vi "Update Refs.vi"(8 "error in (no error)":errorcluster, 10 "SequencerInfo":refnum<class "SequencerInfo.lvclass">, 11 "UI in":refnum<class "UI.lvclass">) -> (0 "error out":errorcluster, 3 "UI out":refnum<class "UI.lvclass">)   [LabVIEW 2015, in "UI.lvlib" / "UI.lvclass"]
uses:
  UI.lvclass
  Sequencer/SequencerInfo.lvclass
  Sequencer/SequencerConfig.lvclass
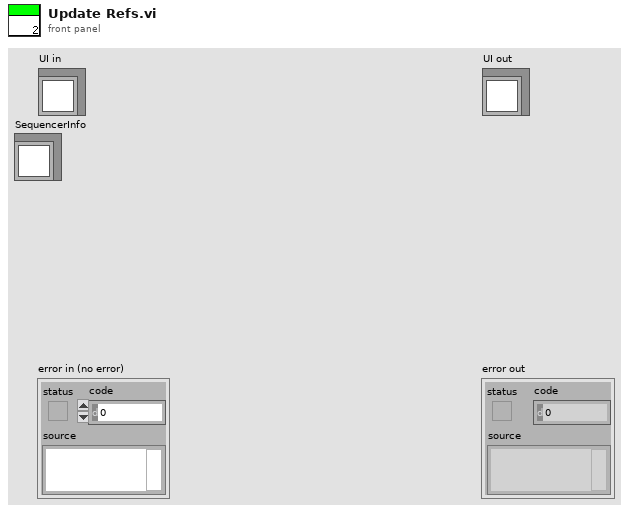
[diagram p1: front panel]
types:
  T1 = typedef "Sequencer.lvlib/Sequencer.lvclass/Daq Channel Info.ctl" = cluster{"DevNames":tag[], "AO.PhysicalChans":tag[][], "DO.Lines":tag[][], "AI.PhysicalChans":tag[][]}
  T2 = cluster{"Accessors:Sample Rate":dbl, "Accessors:Buffer Size":dbl}
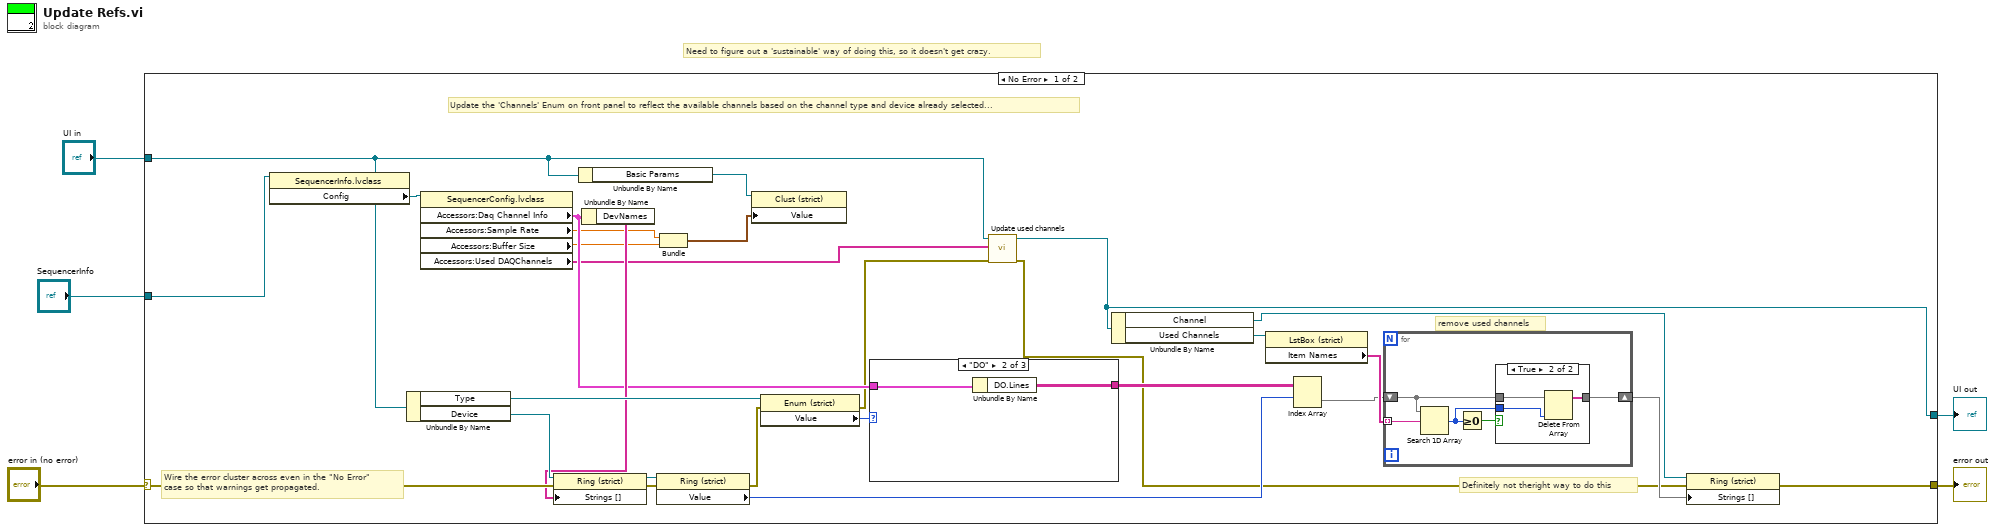
[diagram p0: block diagram]
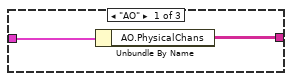
[diagram p3: hidden frame]
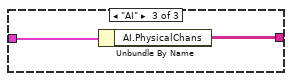
[diagram p4: hidden frame]
diagram:
  # "Need to figure out a 'sustainable' way of doing this, so it doesn't get crazy."
  n1 = case shown="No Error" "error in (no error)" {
    selector: "error in (no error)" -> [w25 w50]
    tunnel: [w14 w50] -> w4
    tunnel: [w8 w49] -> w2
    tunnel: "UI in" -> [w9 w49]
    tunnel: "SequencerInfo" -> [w11 _]
    frame No Error {
      # "Update the 'Channels' Enum on front panel to reflect the available channels based on the channel type and device already selected..."
      # "remove used channels"
      # "Definitely not theright way to do this"
      # "Wire the error cluster across even in the \"No Error\"\ncase so that warnings get propagated."
      n2 = property class="SequencerInfo.lvclass"(reference=w11) -> ("Config"=w19:refnum<class "SequencerConfig.lvclass">)  [unwired: 1 in, 2 out]
      n3 = Unbundle By Name(w9) -> ("Type"=w30:refnum<vi>, "Device"=w33:refnum<vi>)
      n4 = property class="SequencerConfig.lvclass"(reference=w19) -> ("Accessors:Daq Channel Info"=w17:T1, "Accessors:Sample Rate"=w16:dbl, "Accessors:Buffer Size"=w15:dbl, "Accessors:Used DAQChannels"=w10:tag[])  [unwired: 1 in, 2 out]
      n5 = Unbundle By Name(w9) -> ("Basic Params"=w13:refnum<vi>)
      n6 = Unbundle By Name(w17) -> ("DevNames"=w18:tag[])
      n7 = property class="Ring (strict)"(reference=w33, error in=w25, "Strings []"=w18) -> (reference out=w32:refnum<vi>, error out=w31:errorcluster)
      n8 = property class="Ring (strict)"(reference=w32, error in=w31) -> (error out=w26:errorcluster, "Value"=w24:u16)  [unwired: 1 out]
      n9 = Bundle("Accessors:Sample Rate"=w16, "Accessors:Buffer Size"=w15) -> (w12:T2)  [unwired: 1 in]
      n10 = property class="Clust (strict)"(reference=w13, "Value"=w12) -> ()  [unwired: 1 in, 2 out]
      n11 = property class="Enum (strict)"(reference=w30, error in=w26) -> (error out=w7:errorcluster, "Value"=w29:enum16{"AO", "DO", "AI"})  [unwired: 1 out]
      n12 = case shown="\"DO\"" w29 {
        tunnel: [w44 w46 w48] -> w27
        tunnel: w17 -> [w43 w45 w47]
        frame "AO" {
          n13 = Unbundle By Name(w43) -> ("AO.PhysicalChans"=w44:tag[][])
        }
        frame "DO" {
          n14 = Unbundle By Name(w45) -> ("DO.Lines"=w46:tag[][])
        }
        frame "AI" {
          n15 = Unbundle By Name(w47) -> ("AI.PhysicalChans"=w48:tag[][])
        }
      }
      n16 = call "Update used channels.vi"("error in (no error)"=w7, "Used DAQ Channels in"=w10, "UI in"=w9) -> ("error out"=w6:errorcluster, "UI out"=w8:refnum<class "UI.lvclass">)  [unwired: 7 in]
      n17 = Unbundle By Name(w8) -> ("Channel"=w28:refnum<vi>, "Used Channels"=w23:refnum<vi>)
      n18 = property class="LstBox (strict)"(reference=w23) -> ("Item Names"=w22:string[])  [unwired: 1 in, 2 out]
      n19 = Index Array(array=w27, index (row)=w24) -> (element=w21:tag[])  [unwired: 1 in]
      n20 = for {
        tunnel: w22 -> [w38] mode=indexing
        shift-right: [w36] -> w20
        shift-left: w21 -> [w37]
        n21 = Search 1D Array(1D array=w37, element=w38) -> (index of element=w35:i32)  [unwired: 1 in]
        n22 = Greater Or Equal To 0?(x=w35) -> (x >= 0?=w34:bool)
        n23 = case shown="True" w34 {
          tunnel: w37 -> [w39 w42]
          tunnel: w35 -> [_ w41]
          tunnel: [w39 w40] -> w36
          frame False {
          }
          frame True {
            n24 = Delete From Array(array=w42, index=w41) -> (array with subset deleted=w40:tag[])  [unwired: 1 in, 1 out]
          }
        }
      }
      n25 = property class="Ring (strict)"(reference=w28, error in=w6, "Strings []"=w20) -> (error out=w14:errorcluster)  [unwired: 1 out]
    }
    frame Error {
    }
  }
  "error out" <- w4
  "UI out" <- w2
